vi "Next Frame.vi"(11 "Animated Texture in":refnum<class "Animated Texture.lvclass">) -> (3 "Animated Texture out":refnum<class "Animated Texture.lvclass">)   [LabVIEW 2015, in "Animated Texture.lvclass"]
uses:
  Animated Texture.lvclass
  Animated Texture.lvclass/Animated Texture.ctl
panel:
  in  "y":i32
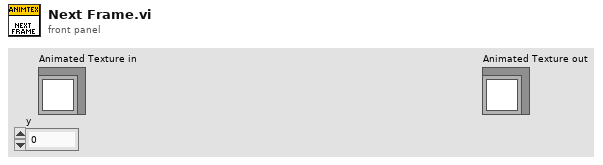
[diagram p1: front panel]
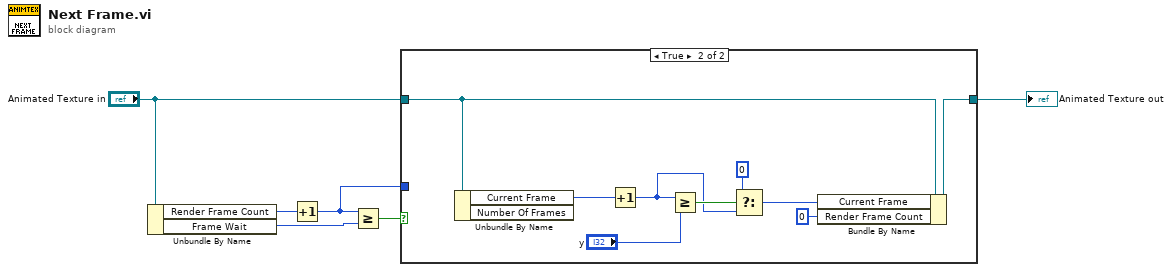
[diagram p0: block diagram]
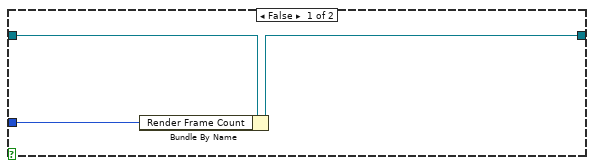
[diagram p2: hidden frame]
diagram:
  n1 = Unbundle By Name("Animated Texture in") -> ("Render Frame Count"=w4:i32, "Frame Wait"=w3:i32)
  n2 = Increment(x=w4) -> (x+1=w1:i32)
  n3 = Greater Or Equal?(x=w1, y=w3) -> (x >= y?=w2:bool)
  n4 = case shown="True" w2 {
    tunnel: [w7 w18] -> w6
    tunnel: "Animated Texture in" -> [w9 w12]
    tunnel: w1 -> [w8 _]
    frame False {
      n5 = Bundle By Name(cluster=w9, "Render Frame Count"=w8) -> (w7:refnum<class "Animated Texture.lvclass">)
    }
    frame True {
      n6 = Unbundle By Name(w12) -> ("Current Frame"=w17:i32)  [unwired: 1 out]
      n7 = Increment(x=w17) -> (x+1=w14:i32)
      n8 = Greater Or Equal?(x=w14, y="y") -> (x >= y?=w16:bool)
      n9 = Select(t=0, s=w16, f=w14) -> (s? t:f=w13:i32)
      n10 = Bundle By Name(cluster=w12, "Current Frame"=w13, "Render Frame Count"=0) -> (w18:refnum<class "Animated Texture.lvclass">)
    }
  }
  "Animated Texture out" <- w6
